vi "dfd_Apply MRate Gain.vi"(10 "multirate filter":T1={"mMRate_Structure"=enum."CIC", "mMRate_Mode"=0, "mMRate_Factor"=1, "mMRate_FIRParams"={"mMRate_FIR_H"=[], "mMRate_FIR_IsNyquist?"=FALSE, "mMRate_FIR_IsSymmetric?"=FALSE}, "mMRate_CICParams"={"mMRate_CIC_#Stage"=2, "mMRate_CIC_Lag"=1, "mMRate_CIC_Type"=enum."Lowpass"}, "mMRate_Order"=0, "mMRate_Version"="1.0", "mMRate_Comments"="", "mMRate_RationalFactor"={"mMRate_L"=-1, "mMRate_M"=-1}, "mMRate_Fs"=1.0, "mMRate_Quantized?"=FALSE, "mMRate_QFilterGain"=1.0, "mMRate_CoefWl"=16, "mMRate_Scaling"={"mMRate_ScaleByPowerOf2?"=FALSE, "mMRate_ScaleType"=enum."Time Domain 1-Norm"}, "mMRate_InputWl"=0, "mMRate_OutputWl"=0, "mMRate_OutputMode"=enum."Nearest", "mMRate_MultMode"=enum."Truncated", "mMRate_BitPruning"=FALSE, "mMRate_GainWl"=16, "mMRate_OutputFwl"=0, "mMRate_SumIwl"=0, "mMRate_InputIwl "=16, "mMRate_SumWl"=32, "mMRate_CoefIwl"=0} {"mMRate_SumWl" min=1 max=32 step=1; "mMRate_InputIwl" min=1 max=32 step=1; "mMRate_GainWl" min=1 max=32 step=1; "mMRate_OutputWl" min=1 max=32 step=1; "mMRate_InputWl" min=1 max=32 step=1; "mMRate_CoefWl" min=1 max=32 step=1; "mMRate_Mode" items=["Default"=-1, "No Rate Change"=0, "Interpolation"=1, "Decimation"=2, "Interpolated"=3, "Rational"=4]}, 11 "signal in":i64[](array[numeric])) -> (3 "signal out":i64[](array[numeric]))   [LabVIEW 2017, in "NI_DigFilter_FXP.lvlib"]
uses:
  <vilib>/addons/Digital Filter Design/NI_DigFilter_FXP.lvlib
  <vilib>/addons/Digital Filter Design/_Objects.llb/DFD Multirate Filter Obj.ctl
  <vilib>/addons/Digital Filter Design/_Objects.llb/DFD Multirate Mode.ctl
  <vilib>/addons/Digital Filter Design/_Objects.llb/DFD Coef Norm Type.ctl
  <vilib>/addons/Digital Filter Design/_Objects.llb/DFD Round-off Mode.ctl
  <vilib>/addons/Digital Filter Design/_Objects.llb/DFD FXP MRate Multiply Mode.ctl
  <vilib>/addons/Digital Filter Design/NI_DigFilterLicensed.lvlib
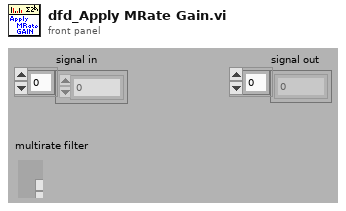
[diagram p1: front panel]
types:
  T1 = typedef "NI_DigFilterLicensed.lvlib/DFD Multirate Filter Obj.ctl" = cluster{"mMRate_Structure":enum16{"CIC", "FIR", "IIR", "Lattice"}, "mMRate_Mode":T2, "mMRate_Factor":i32, "mMRate_FIRParams":cluster{"mMRate_FIR_H":dbl[], "mMRate_FIR_IsNyquist?":bool, "mMRate_FIR_IsSymmetric?":bool}, "mMRate_CICParams":cluster{"mMRate_CIC_#Stage":i32, "mMRate_CIC_Lag":i32, "mMRate_CIC_Type":enum16{"Lowpass", "Highpass"}}, "mMRate_Order":i32, "mMRate_Version":string, "mMRate_Comments":string, "mMRate_RationalFactor":cluster{"mMRate_L":i32, "mMRate_M":i32}, "mMRate_Fs":dbl, "mMRate_Quantized?":bool, "mMRate_QFilterGain":dbl, "mMRate_CoefWl":i16, "mMRate_Scaling":cluster{"mMRate_ScaleByPowerOf2?":bool, "mMRate_ScaleType":T3}, "mMRate_InputWl":i16, "mMRate_OutputWl":i16, "mMRate_OutputMode":T4, "mMRate_MultMode":T5, "mMRate_BitPruning":bool, "mMRate_GainWl":i16, "mMRate_OutputFwl":i16, "mMRate_SumIwl":i16, "mMRate_InputIwl ":i16, "mMRate_SumWl":i16, "mMRate_CoefIwl":i16}
  T2 = typedef "NI_DigFilterLicensed.lvlib/DFD Multirate Mode.ctl" = i16
  T3 = typedef "NI_DigFilterLicensed.lvlib/DFD Coef Norm Type.ctl" = enum16{"No Norm", "Time Domain 1-Norm", "Time Domain 2-Norm", "Time Domain Inf-Norm"}
  T4 = typedef "NI_DigFilterLicensed.lvlib/DFD Round-off Mode.ctl" = enum16{"Nearest", "Truncation"}
  T5 = typedef "NI_DigFilterLicensed.lvlib/DFD FXP MRate Multiply Mode.ctl" = enum16{"Truncated", "Full"}
  T6 = typedef "NI_DigFilterLicensed.lvlib/dfd_Internal Quantization Settings.ctl" = cluster{"source":T7, "wl":i16, "iwl":i16, "overflow mode":enum16{"Saturation", "Wrap"}, "rounding mode":enum16{"Nearest", "Truncation"}, "signed?":bool}
  T7 = typedef "NI_DigFilterLicensed.lvlib/dfd_Internal Quantization Srcs.ctl" = u16
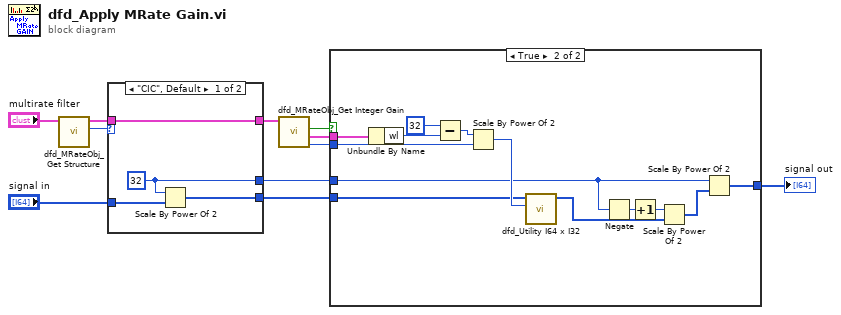
[diagram p0: block diagram]
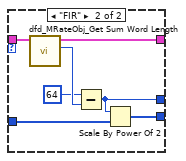
[diagram p2: hidden frame]
diagram:
  n1 = call <vilib>:"dfd_MRateObj_Get Structure.vi"("multirate filter in"="multirate filter") -> ("structure"=w5:enum16{"CIC", "FIR", "IIR", "Lattice"}, "dup multirate filter"=w4:T1)  [unwired: 9 out]
  n2 = case shown="\"CIC\", Default" w5 {
    tunnel: "signal in" -> [w15 w19]
    tunnel: w4 -> [w12 w22]
    tunnel: [w14 w18] -> w3
    tunnel: [w13 w17] -> w2
    tunnel: [w12 w16] -> w1
    frame "CIC", Default {
      w13 = i16 32 ("n")
      n3 = Scale By Power Of 2(n=w13, x=w15) -> (x*2^n=w14:i64[])
    }
    frame "FIR" {
      n4 = call <vilib>:"dfd_MRateObj_Get Sum Word Length.vi"("multirate filter in"=w22) -> ("SumWl"=w21:i16, "multirate filter out"=w16:T1)  [unwired: 9 out]
      n5 = Subtract(x=i16 64, y=w21) -> (x-y=w17:i16)
      n6 = Scale By Power Of 2(n=w17, x=w19) -> (x*2^n=w18:i64[])
    }
  }
  n7 = call <vilib>:"dfd_MRateObj_Get Integer Gain.vi"("multirate filter"=w1) -> ("I32 gain"=w10:i32, "Gain quantizer"=w11:T6, "on FPGA?"=w9:bool)  [unwired: 8 out]
  n8 = case shown="True" w9 {
    tunnel: w3 -> [w23 w30]
    tunnel: [w23 w27] -> w8
    tunnel: w11 -> [_ w36]
    tunnel: w10 -> [_ w35]
    tunnel: w2 -> [_ w26]
    frame False {
    }
    frame True {
      n9 = Unbundle By Name(w36) -> ("wl"=w34:i16)
      n10 = Subtract(x=i16 32, y=w34) -> (x-y=w32:i16)
      n11 = Scale By Power Of 2(n=w32, x=w35) -> (x*2^n=w31:i32)
      n12 = call <vilib>:"dfd_Utility I64 x I32 .vi"("y[I32]"=w31, "x[I64]"=w30) -> ("x*y[Hi I64]"=w24:i64[])  [unwired: 9 out]
      n13 = Negate(x=w26) -> (-x=w29:i16)
      n14 = Increment(x=w29) -> (x+1=w25:i16)
      n15 = Scale By Power Of 2(n=w25, x=w24) -> (x*2^n=w28:i64[])
      n16 = Scale By Power Of 2(n=w26, x=w28) -> (x*2^n=w27:i64[])
    }
  }
  "signal out" <- w8
